vi "读excel程序（OK）.vi"(4 "路径":path) -> (1 "数组":string[][](array[string]))   [LabVIEW 2014]
panel:
  out "错误输出":errorcluster
  in  "自动化引用句柄输入":refnum<k7>
  in  "Excel._Application":refnum<k7>
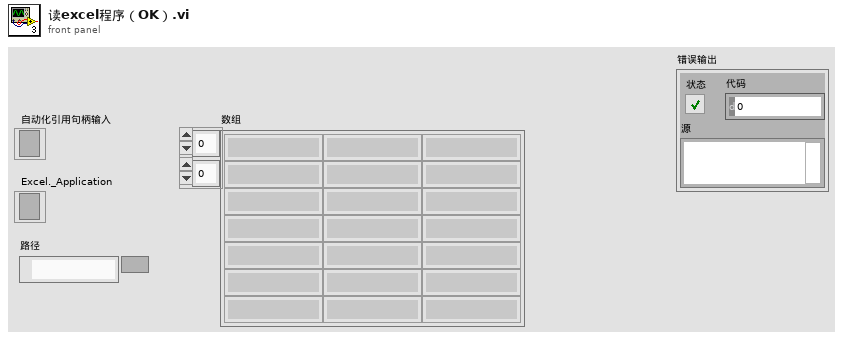
[diagram p1: front panel]
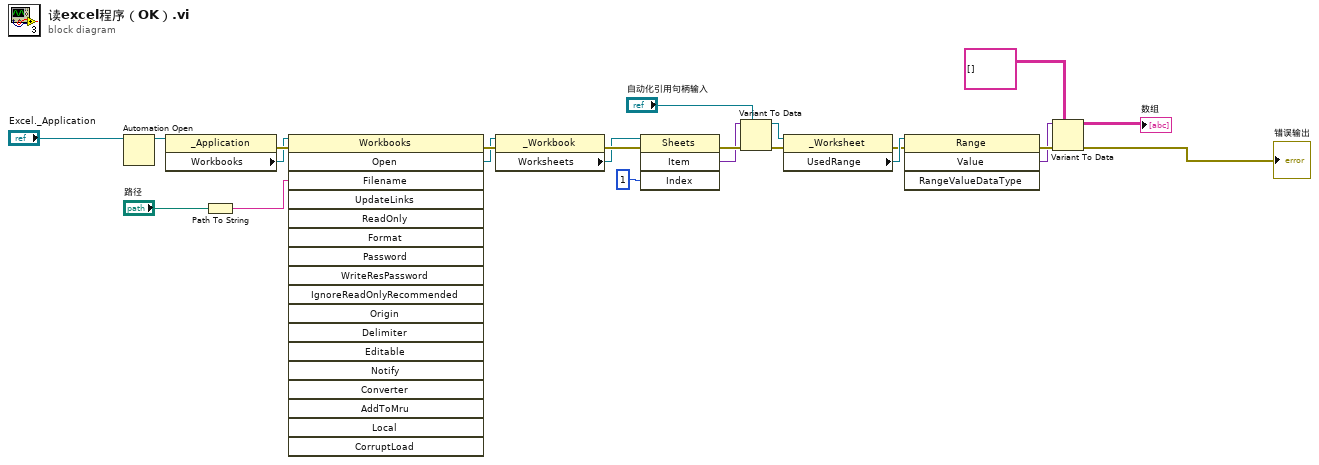
[diagram p0: block diagram]
diagram:
  n1 = Automation Open(Automation Refnum="Excel._Application") -> (Automation Refnum=w3:refnum<k7>)  [unwired: 3 in, 1 out]
  n2 = property on="属性节点" class="_Application"(reference=w3) -> (error out=w5:errorcluster, "Workbooks"=w4:refnum<k7>)  [unwired: 1 in, 1 out]
  n3 = Path To String(path="路径") -> (string=w7:string)
  n4 = invoke class="Workbooks" method="Open"(reference=w4, error in=w5, "Filename"=w7) -> (error out=w9:errorcluster, "Open"=w8:refnum<k7>)  [unwired: 15 in, 16 out]
  n5 = property class="_Workbook"(reference=w8, error in=w9) -> (error out=w11:errorcluster, "Worksheets"=w10:refnum<k7>)  [unwired: 1 out]
  n6 = invoke class="Sheets" method="Item"(reference=w10, error in=w11, "Index"=1) -> (error out=w14:errorcluster, "Item"=w13:variant)  [unwired: 1 in, 2 out]
  n7 = Variant To Data(error in=w14, type="自动化引用句柄输入", Variant=w13) -> (data=w17:refnum<k7>, error out=w16:errorcluster)
  n8 = property class="_Worksheet"(reference=w17, error in=w16) -> (error out=w18:errorcluster, "UsedRange"=w19:refnum<k7>)  [unwired: 1 out]
  n9 = invoke class="Range" method="Value"(reference=w19, error in=w18) -> (error out=w21:errorcluster, "Value"=w20:variant)  [unwired: 2 in, 2 out]
  n10 = Variant To Data(error in=w21, type=string[][] [], Variant=w20) -> (data=→"数组":string[][], error out=→"错误输出":errorcluster)
